vi "Get Version Info.vi"(9 "ui32BufferLen":u32, 10 "szVersionInfo":string, 11 "arr":u32(ring)=65535 items=["AT_SDKVersion"=1073741824, "AT_DeviceDriverVersion"=1073741825]) -> (2 "szVersionInfo out":string, 3 "function return":u32)   [LabVIEW 2018, in "AndorSDK.lvlib"]
doc: "EXPNETTYPE unsigned int WINAPI GetVersionInfo(AT_VersionInfoId arr, char * szVersionInfo, at_u32 ui32BufferLen);"
uses:
  AndorSDK.lvlib
  ATMCD32D.dll
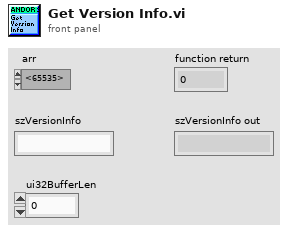
[diagram p1: front panel]
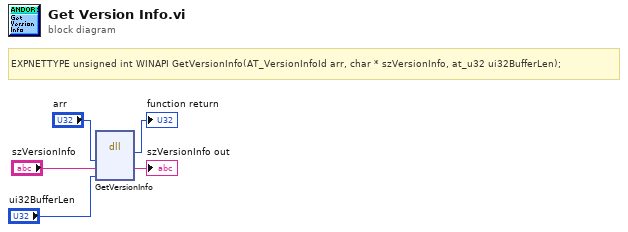
[diagram p0: block diagram]
diagram:
  # "EXPNETTYPE unsigned int WINAPI GetVersionInfo(AT_VersionInfoId arr, char * szVersionInfo, at_u32 ui32BufferLen);"
  n1 = dll-call lib="PTH2babs E\nPersönliches02 - Arbeit03-HiwijobsLabviewCodelibANDOR\tAndor SDK\nATMCD32D.*" fn="GetVersionInfo"("arr"="arr", "szVersionInfo"="szVersionInfo", "ui32BufferLen"="ui32BufferLen") -> (→"function return":u32, "szVersionInfo"=→"szVersionInfo out":string)  [unwired: 5 in, 2 out]
